vi "measureCombs_anySet2.vi"(3 "Read freqs. \nfrom textfile":bool, 5 "Cluster":T2={"span"=200000000.0, "rbw"=1000.0, "enableVBW"=FALSE, "vbw"=0.0, "traceLength"=64001, "window"=0, "verticalUnit"=0, "center freq"=100000000.0} {"verticalUnit" items=["SpectrumVerticalUnit_dBm", "SpectrumVerticalUnit_Watt", "SpectrumVerticalUnit_Volt", "SpectrumVerticalUnit_Amp", "SpectrumVerticalUnit_dBmV"]; "window" items=["SpectrumWindow_Kaiser", "SpectrumWindow_Mil6dB", "SpectrumWindow_BlackmanHarris", "SpectrumWindow_Rectangle", "SpectrumWindow_FlatTop", "SpectrumWindow_Hann"]; "traceLength" items=["801"=801, "2401"=2401, "4001"=4001, "8001"=8001, "10401"=10401, "16001"=16001, "32001"=32001, "64001"=64001]}, 6 "error in":errorcluster, 7 "Burn time/ RFC measurement time":i32=2, 8 "AFC & OFC Measurement time":i32=2, 9 "Folder for all data (Don't forget the last slash!)":string="C:\\Users\\Lab\\Desktop\\Data\\2019-08\\2019-08-07\\") -> (0 "error out":errorcluster)   [LabVIEW 2016]
uses:
  <vilib>/Utility/file.llb/Read Delimited Spreadsheet (DBL).vi
  <vilib>/Utility/file.llb/Write Delimited Spreadsheet (DBL).vi
panel:
  in  "stop":bool
  out "error out 2":errorcluster
  out "traceData out":sgl[](graph)
  out "To change these settings, you must edit them in the block diagram":T1(array[cluster])
  in  "Sweep probe twice":bool
  out "Current set #":i32
  out "Current freq.":dbl
  in  "freqs. file":path
  in  "Shuffle?":bool
  in  "Start freq":dbl=1000000.0 format="%0.2e"
  in  "End freq":dbl=2000000.0 format="%0.2e"
  in  "Freq step":i32=100000 format="%.2e"
  out "Duration array":T3(array[cluster])
  in  "Mod shape":enum16{"Triangle", "Sine"}(ring)
  # "consecutive sweeps can be compared\nto check for probe on AFC."
  # "RSA settings"
  # "Suppose you want to collect comb data, first ascending, then descending.\n\nIn Matlab, create a 1xM array \ncontaining all modulation freqs (Hz) in the ascending sequence; then create a 1xN array for the descending case. Note that M != N is fine.\n\nfid= fopen(FILENAME, 'w');\nfprintf(fid,'%d\\t', ARRAY1);\nfprintf(fid,'\\r\\n');\nfprintf(fid,'%d\\t',ARRAY2);\n... \n(for more sets, repeat as needed)\nfclose(fid);\n\nNow find the file you just made:"
  # "Modulation settings"
  # "(zero-indexed)"
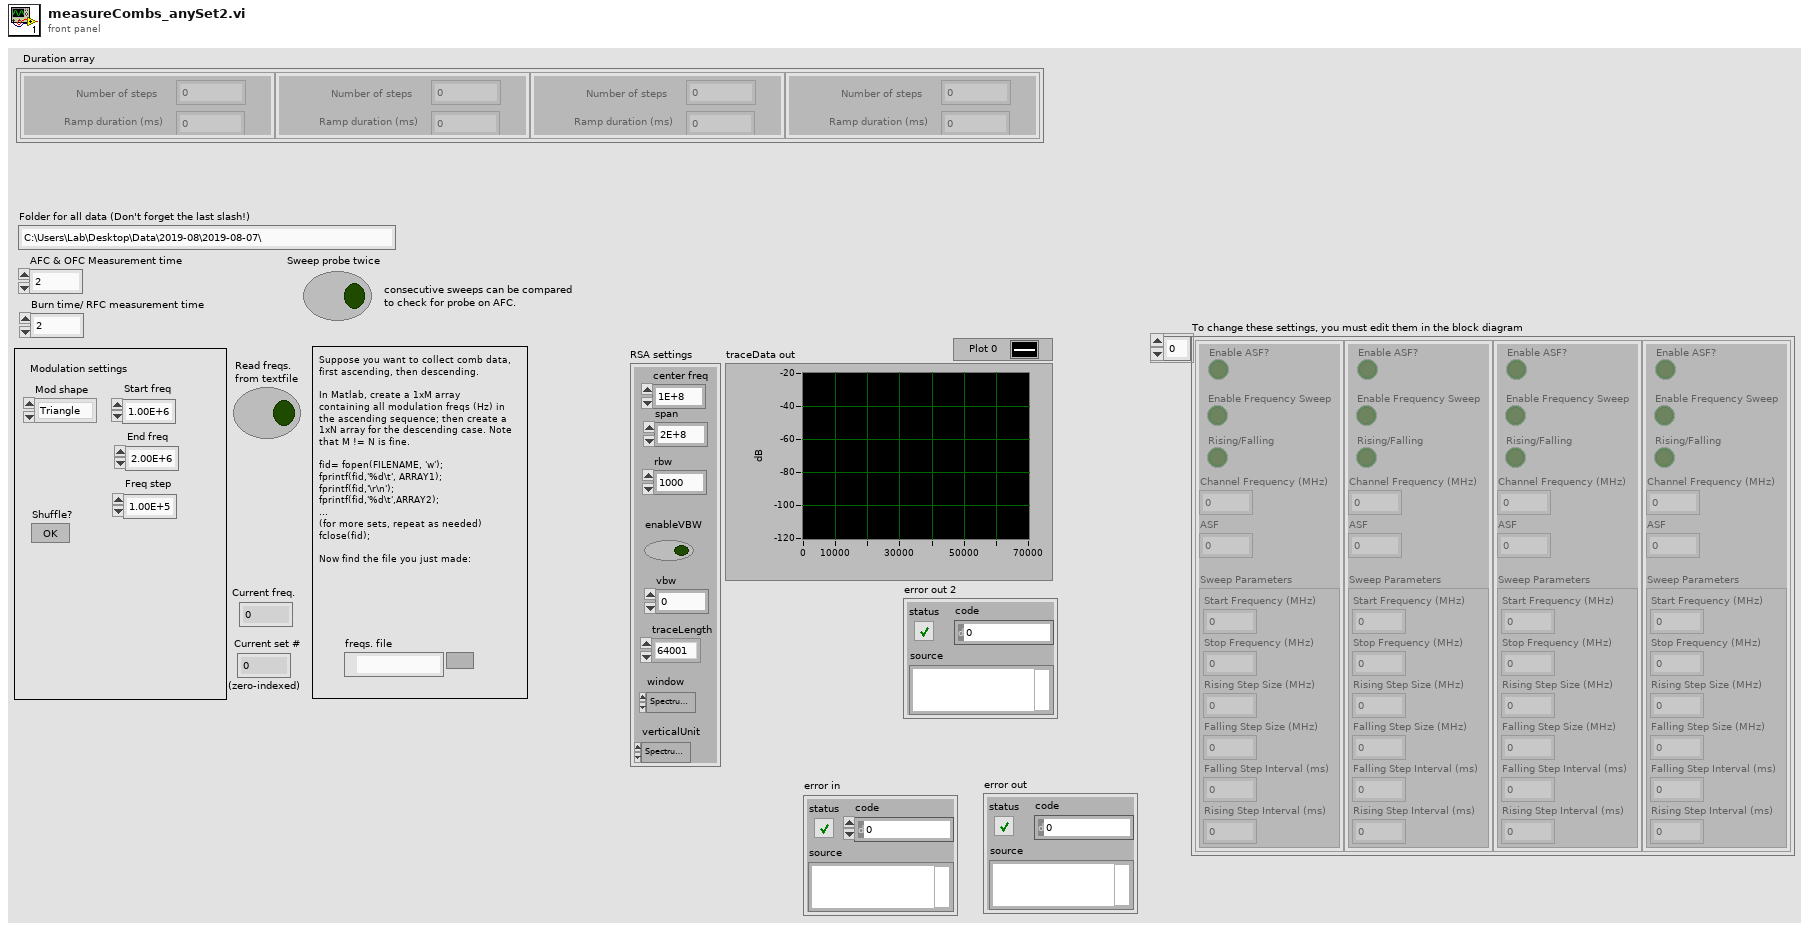
[diagram p1: front panel]
types:
  T1 = cluster{"Enable ASF?":bool, "Channel Frequency (MHz)":dbl, "ASF":dbl, "Enable Frequency Sweep":bool, "Sweep Parameters":cluster{"Start Frequency (MHz)":dbl, "Stop Frequency (MHz)":dbl, "Rising Step Size (MHz)":dbl, "Falling Step Size (MHz)":dbl, "Falling Step Interval (ms)":dbl, "Rising Step Interval (ms)":dbl}, "Rising/Falling":bool}[]
  T2 = cluster{"span":dbl, "rbw":dbl, "enableVBW":bool, "vbw":dbl, "traceLength":u16, "window":u32, "verticalUnit":u32, "center freq":dbl}
  T3 = cluster{"Number of steps":dbl, "Ramp duration (ms)":dbl}[]
  T4 = cluster{"span":dbl, "rbw":dbl, "enableVBW":bool, "vbw":dbl, "traceLength":u16, "window":u32, "verticalUnit":u32}
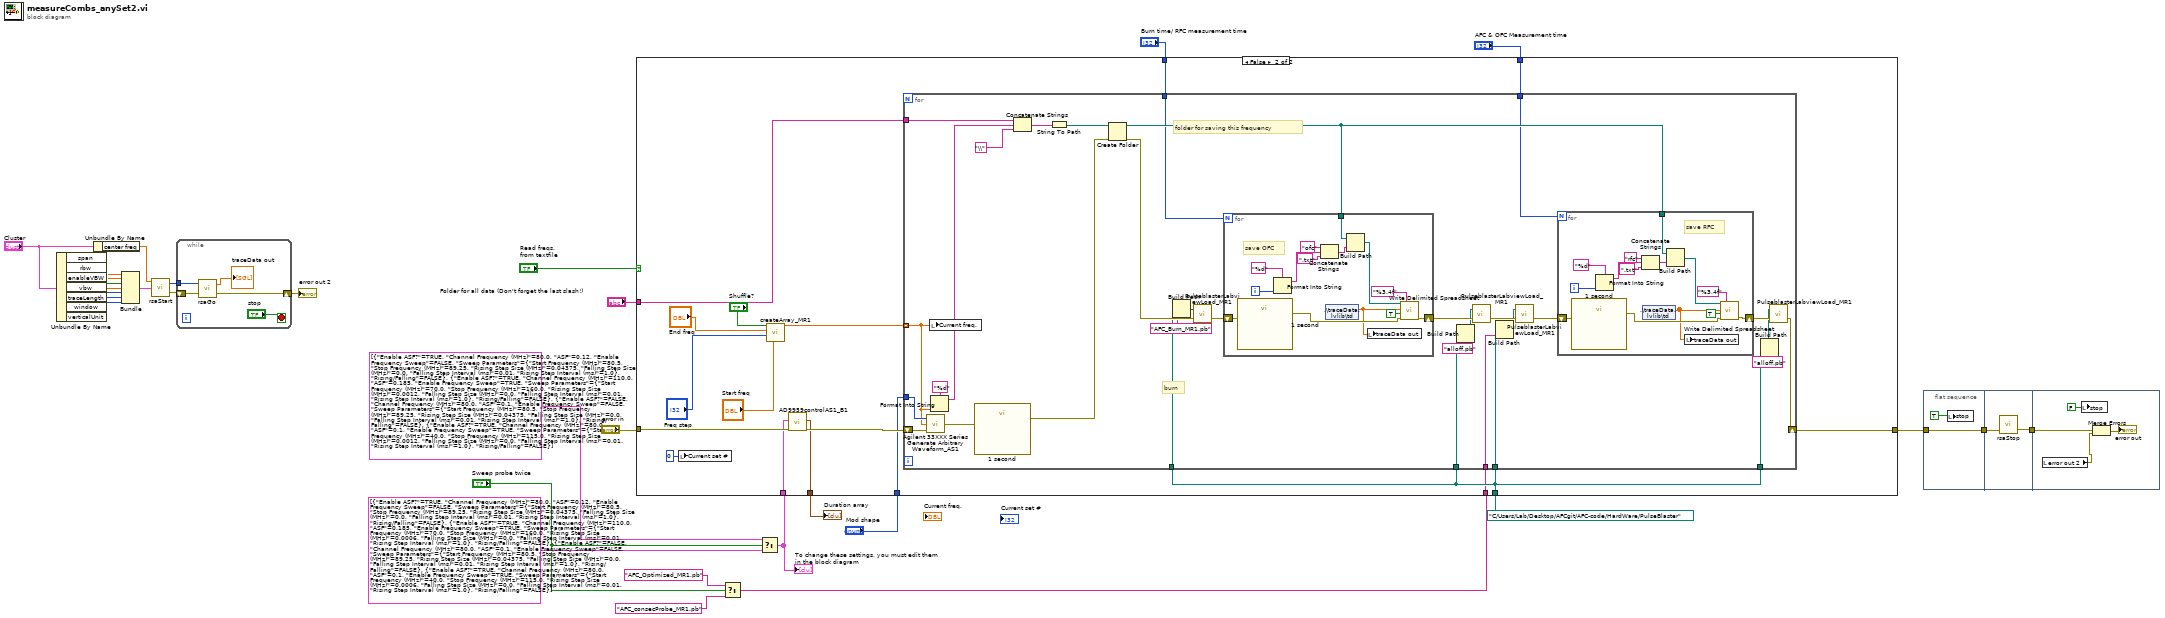
[diagram p0: block diagram]
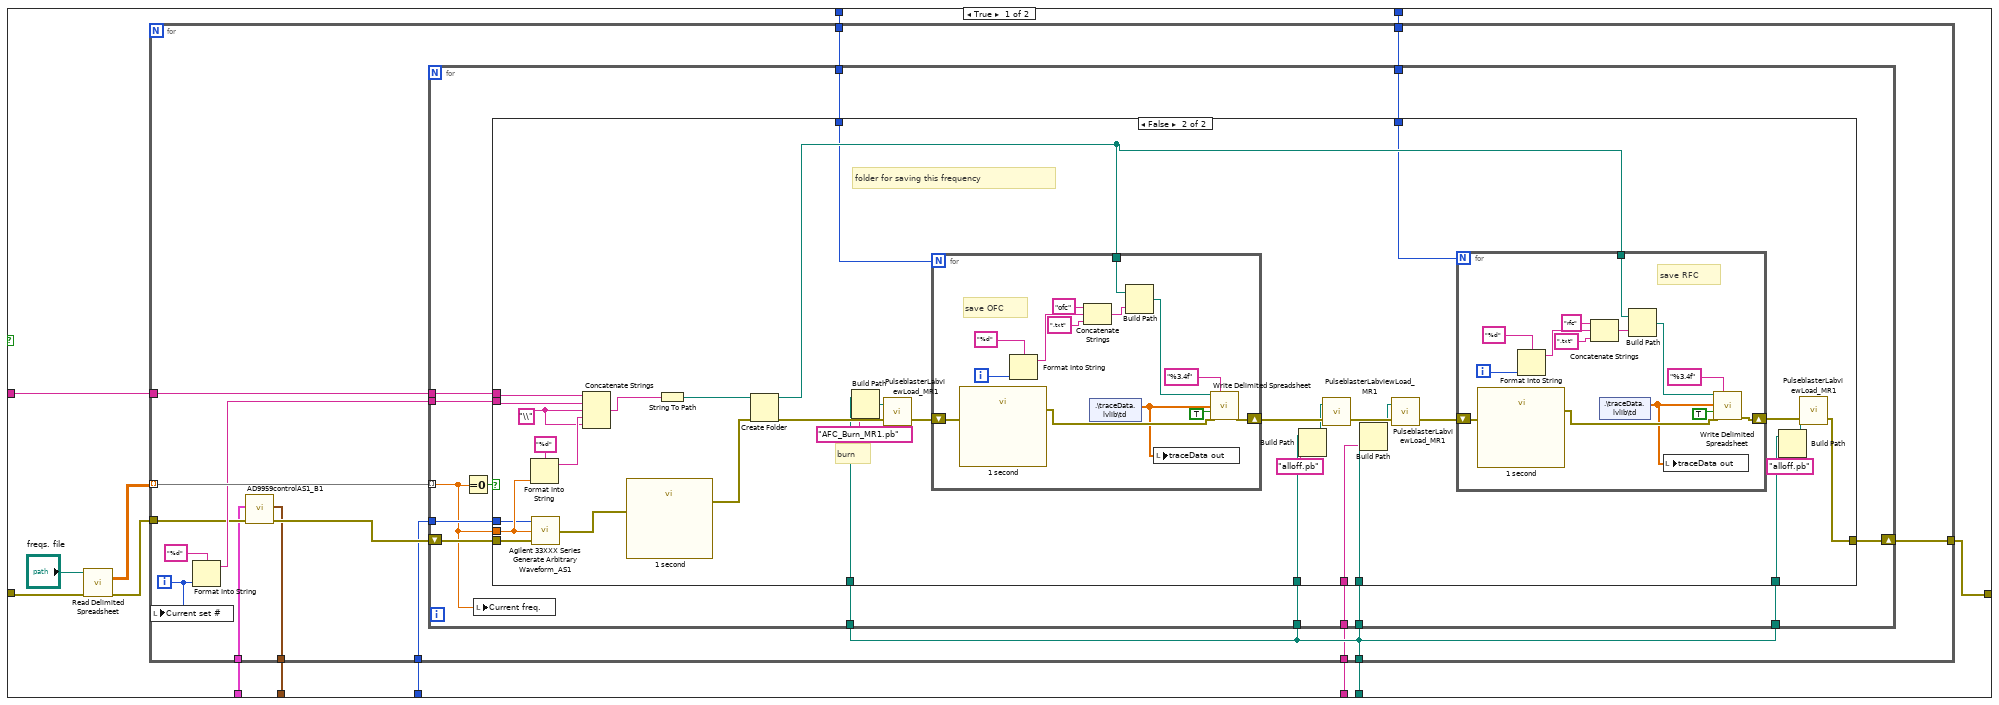
[diagram p2: hidden frame]
diagram:
  n1 = Unbundle By Name("Cluster") -> ("span"=w24:dbl, "rbw"=w25:dbl, "enableVBW"=w26:bool, "vbw"=w27:dbl, "traceLength"=w28:u16, "window"=w29:u32, "verticalUnit"=w30:u32)
  n2 = Unbundle By Name("Cluster") -> ("center freq"=w7:dbl)
  n3 = Bundle("span"=w24, "rbw"=w25, "enableVBW"=w26, "vbw"=w27, "traceLength"=w28, "window"=w29, "verticalUnit"=w30) -> (w6:T4)  [unwired: 1 in]
  n4 = call "rsaStart.vi"("Cluster"=w6, "center freq"=w7) -> ("error out"=w4:errorcluster, "traceLength"=w5:u16)  [unwired: 1 in]
  n5 = while {
    tunnel: w5 -> [w36]
    shift-right: [w34] -> w3
    shift-left: w4 -> [w33]
    stop <- "stop" stop-if-true
    n6 = call "rsaGo.vi"("error in"=w33, "Trace length"=w36) -> ("error out"=w34:errorcluster, "traceData out"=→"traceData out":sgl[])  [unwired: 1 in]
  }
  "error out 2" <- w3
  n7 = Select(t="AFC_Optimized_MR1.pb" ("name or relative path"), s="Sweep probe twice", f="AFC_consecProbe_MR1.pb" ("name or relative path")) -> (s? t:f=w8:string)
  n8 = Select(t=T1 [{"Enable ASF?"=TRUE, "Channel Frequency (MHz)"=80.0, "ASF"=0.12, "Enable Frequency Sweep"=FALSE, "Sweep Parameters"={"Start Frequency (MHz)"=80.5, "Stop Frequency (MHz)"=89.25, "Rising Step Size (MHz)"=0.04375, "Falling Step Size (MHz)"=0.0, "Falling Step Interval (ms)"=0.01, "Rising Step Interval (ms)"=1.0}, "Rising/Falling"=FALSE}, {"Enable ASF?"=TRUE, "Channel Frequency (MHz)"=110.0, "ASF"=0.185, "Enable Frequency Sweep"=TRUE, "Sweep Parameters"={"Start Frequency (MHz)"=70.0, "Stop Frequency (MHz)"=160.0, "Rising Step Size (MHz)"=0.0012, "Falling Step Size (MHz)"=0.0, "Falling Step Interval (ms)"=0.01, "Rising Step Interval (ms)"=1.0}, "Rising/Falling"=FALSE}, {"Enable ASF?"=FALSE, "Channel Frequency (MHz)"=80.0, "ASF"=0.1, "Enable Frequency Sweep"=FALSE, "Sweep Parameters"={"Start Frequency (MHz)"=80.5, "Stop Frequency (MHz)"=89.25, "Rising Step Size (MHz)"=0.04375, "Falling Step Size (MHz)"=0.0, "Falling Step Interval (ms)"=0.01, "Rising Step Interval (ms)"=1.0}, "Rising/Falling"=FALSE}, {"Enable ASF?"=TRUE, "Channel Frequency (MHz)"=80.0, "ASF"=0.1, "Enable Frequency Sweep"=TRUE, "Sweep Parameters"={"Start Frequency (MHz)"=40.0, "Stop Frequency (MHz)"=115.0, "Rising Step Size (MHz)"=0.0012, "Falling Step Size (MHz)"=0.0, "Falling Step Interval (ms)"=0.01, "Rising Step Interval (ms)"=1.0}, "Rising/Falling"=FALSE}] ("Array"), s="Sweep probe twice", f=T1 [{"Enable ASF?"=TRUE, "Channel Frequency (MHz)"=80.0, "ASF"=0.12, "Enable Frequency Sweep"=FALSE, "Sweep Parameters"={"Start Frequency (MHz)"=80.5, "Stop Frequency (MHz)"=89.25, "Rising Step Size (MHz)"=0.04375, "Falling Step Size (MHz)"=0.0, "Falling Step Interval (ms)"=0.01, "Rising Step Interval (ms)"=1.0}, "Rising/Falling"=FALSE}, {"Enable ASF?"=TRUE, "Channel Frequency (MHz)"=110.0, "ASF"=0.185, "Enable Frequency Sweep"=TRUE, "Sweep Parameters"={"Start Frequency (MHz)"=70.0, "Stop Frequency (MHz)"=160.0, "Rising Step Size (MHz)"=0.0006, "Falling Step Size (MHz)"=0.0, "Falling Step Interval (ms)"=0.01, "Rising Step Interval (ms)"=1.0}, "Rising/Falling"=FALSE}, {"Enable ASF?"=FALSE, "Channel Frequency (MHz)"=80.0, "ASF"=0.1, "Enable Frequency Sweep"=FALSE, "Sweep Parameters"={"Start Frequency (MHz)"=80.5, "Stop Frequency (MHz)"=89.25, "Rising Step Size (MHz)"=0.04375, "Falling Step Size (MHz)"=0.0, "Falling Step Interval (ms)"=0.01, "Rising Step Interval (ms)"=1.0}, "Rising/Falling"=FALSE}, {"Enable ASF?"=TRUE, "Channel Frequency (MHz)"=80.0, "ASF"=0.1, "Enable Frequency Sweep"=TRUE, "Sweep Parameters"={"Start Frequency (MHz)"=40.0, "Stop Frequency (MHz)"=115.0, "Rising Step Size (MHz)"=0.0006, "Falling Step Size (MHz)"=0.0, "Falling Step Interval (ms)"=0.01, "Rising Step Interval (ms)"=1.0}, "Rising/Falling"=FALSE}] ("Array")) -> (s? t:f=w12:T1)
  "To change these settings, you must edit them in the block diagram" <- w12
  n9 = case shown="False" "Read freqs. \nfrom textfile" {
    tunnel: "Folder for all data (Don't forget the last slash!)" -> [w49 w158]
    tunnel: path "C:/Users/Lab/Desktop/AFCgit/AFC-code/HardWare/PulseBlaster" ("base path") -> [w39 w157]
    tunnel: "Burn time/ RFC measurement time" -> [w48 w155]
    tunnel: "AFC & OFC Measurement time" -> [w47 w154]
    tunnel: "error in" -> [w45 w148]
    tunnel: "Mod shape" -> [w42 w147]
    tunnel: w12 -> [w41 w146]
    tunnel: [w40 w145] -> w15
    tunnel: w8 -> [w38 w143]
    tunnel: [w37 w142] -> w31
    frame True {
      n10 = call-poly <vilib>:"Read Delimited Spreadsheet.vi"("file path (dialog if empty)"="freqs. file", "error in (no error)"=w45) -> ("all rows"=w44:dbl[][], "error out"=w43:errorcluster)  [unwired: 8 in, 4 out]
      n11 = for {
        tunnel: [w64] -> w37
        tunnel: w49 -> [w63]
        tunnel: w39 -> [w62]
        tunnel: w48 -> [w60]
        tunnel: w47 -> [w59]
        tunnel: w44 -> [w58] mode=indexing
        tunnel: w43 -> [w55]
        tunnel: w42 -> [w54]
        tunnel: w41 -> [w53]
        tunnel: [w52] -> w40
        tunnel: w38 -> [w50]
        i -> [w51]
        n12 = local write "Current set #"(w51) -> ()
        n13 = Format Into String(format string="%d", w51) -> (resulting string=w56:string)  [unwired: 2 in, 1 out]
        n14 = call "AD9959controlAS1_B1.vi"("error in (no error)"=w55, "Array"=w53) -> ("error out"=w61:errorcluster, "Duration array"=w52:T3)  [unwired: 8 in]
        n15 = for {
          tunnel: w58 -> [w66] mode=indexing
          tunnel: w54 -> [w78]
          shift-right: [w77] -> w64
          shift-left: w61 -> [w76]
          tunnel: w63 -> [w68]
          tunnel: w62 -> [w75]
          tunnel: w62 -> [w74]
          tunnel: w62 -> [w73]
          tunnel: w62 -> [w72]
          tunnel: w60 -> [w71]
          tunnel: w59 -> [w70]
          tunnel: w56 -> [w69]
          tunnel: w50 -> [w65]
          n16 = Equal To 0?(x=w66) -> (x = 0?=w67:bool)
          n17 = local write "Current freq."(w66) -> ()
          n18 = case shown="False" w67 {
            tunnel: w78 -> [_ w81]
            tunnel: [w79 w113] -> w77
            tunnel: w76 -> [w79 w83]
            tunnel: w75 -> [_ w102]
            tunnel: w74 -> [_ w99]
            tunnel: w73 -> [_ w97]
            tunnel: w72 -> [_ w94]
            tunnel: w71 -> [_ w92]
            tunnel: w70 -> [_ w91]
            tunnel: w69 -> [_ w86]
            tunnel: w68 -> [_ w87]
            tunnel: w66 -> [_ w82]
            tunnel: w65 -> [_ w80]
            frame True {
            }
            frame False {
              w89 = "\\" ("string")
              # "folder for saving this frequency"
              # "burn"
              n19 = Format Into String(format string="%d", w82) -> (resulting string=w90:string)  [unwired: 2 in, 1 out]
              n20 = call "Agilent 33XXX Series Generate Arbitrary Waveform_AS1.vi"("error in (no error)"=w83, "Frequency (1000 Hz)"=w82, "Enum"=w81) -> ("error out"=w84:errorcluster)
              n21 = Concatenate Strings(w87, w86, w89, w90, w89) -> (w85:string)
              n22 = call "1 second"("error in (no error)"=w84) -> ("error out"=w106:errorcluster)  [unwired: 10 in]
              n23 = String To Path(string=w85) -> (path=w103:path)
              n24 = Create Folder(path (use dialog)=w103, error in=w106) -> (created path=w104:path, error out=w105:errorcluster)  [unwired: 1 in, 1 out]
              n25 = Build Path(base path=w102, name or relative path="AFC_Burn_MR1.pb") -> (appended path=w100:path)
              n26 = call "PulseblasterLabviewLoad_MR1.vi"("error in (no error)"=w105, "Input file"=w100) -> ("error out"=w112:errorcluster)  [unwired: 1 out]
              n27 = for {
                N: w92 -> [_]
                shift-right: [w140] -> w107
                shift-left: w112 -> [w130]
                tunnel: w104 -> [w133]
                i -> [w131]
                # "save OFC"
                n28 = call "1 second"("error in (no error)"=w130) -> ("error out"=w129:errorcluster)  [unwired: 10 in]
                n29 = Format Into String(format string="%d", w131) -> (resulting string=w136:string)  [unwired: 2 in, 1 out]
                n30 = Concatenate Strings("ofc" ("string"), w136, ".txt" ("string")) -> (w135:string)
                n31 = shared-variable ".\\traceData.lvlib\\td"() -> (w128:dbl[])  [unwired: 1 in, 1 out]
                n32 = Build Path(base path=w133, name or relative path=w135) -> (appended path=w139:path)
                n33 = local write "traceData out"(w128) -> ()
                n34 = call-poly <vilib>:"Write Delimited Spreadsheet.vi"("file path (dialog if empty)"=w139, "format (%.3f)"="%3.4f", "1D data"=w128, "append to file? (new file:F)"=TRUE, "error in (no error)"=w129) -> ("error out"=w140:errorcluster)  [unwired: 9 in, 1 out]
              }
              n35 = Build Path(base path=w97, name or relative path="alloff.pb") -> (appended path=w96:path)
              n36 = call "PulseblasterLabviewLoad_MR1.vi"("error in (no error)"=w107, "Input file"=w96) -> ("error out"=w108:errorcluster)  [unwired: 1 out]
              n37 = Build Path(base path=w99, name or relative path=w80) -> (appended path=w98:path)
              n38 = call "PulseblasterLabviewLoad_MR1.vi"("error in (no error)"=w108, "Input file"=w98) -> ("error out"=w110:errorcluster)  [unwired: 1 out]
              n39 = for {
                N: w91 -> [_]
                shift-right: [w126] -> w109
                shift-left: w110 -> [w116]
                tunnel: w104 -> [w118]
                i -> [w122]
                # "save RFC"
                n40 = call "1 second"("error in (no error)"=w116) -> ("error out"=w115:errorcluster)  [unwired: 10 in]
                n41 = Format Into String(format string="%d", w122) -> (resulting string=w121:string)  [unwired: 2 in, 1 out]
                n42 = Concatenate Strings("rfc" ("string"), w121, ".txt" ("string")) -> (w120:string)
                n43 = shared-variable ".\\traceData.lvlib\\td"() -> (w114:dbl[])  [unwired: 1 in, 1 out]
                n44 = Build Path(base path=w118, name or relative path=w120) -> (appended path=w125:path)
                n45 = local write "traceData out"(w114) -> ()
                n46 = call-poly <vilib>:"Write Delimited Spreadsheet.vi"("file path (dialog if empty)"=w125, "format (%.3f)"="%3.4f", "1D data"=w114, "append to file? (new file:F)"=TRUE, "error in (no error)"=w115) -> ("error out"=w126:errorcluster)  [unwired: 9 in, 1 out]
              }
              n47 = Build Path(base path=w94, name or relative path="alloff.pb") -> (appended path=w93:path)
              n48 = call "PulseblasterLabviewLoad_MR1.vi"("error in (no error)"=w109, "Input file"=w93) -> ("error out"=w113:errorcluster)  [unwired: 1 out]
            }
          }
        }
      }
    }
    frame False {
      n49 = local write "Current set #"(0 ("Current set #")) -> ()
      n50 = call "createArray_MR1.vi"("Start freq"="Start freq", "Freq step"="Freq step", "End freq"="End freq", "Shuffle?"="Shuffle?") -> ("Riffled {X}"=w149:dbl[])  [unwired: 7 in]
      n51 = call "AD9959controlAS1_B1.vi"("error in (no error)"=w148, "Array"=w146) -> ("error out"=w156:errorcluster, "Duration array"=w145:T3)  [unwired: 8 in]
      n52 = for {
        tunnel: w149 -> [w161] mode=indexing
        tunnel: w147 -> [w191]
        shift-right: [w190] -> w142
        shift-left: w156 -> [w189]
        tunnel: w158 -> [w164]
        tunnel: w157 -> [w174]
        tunnel: w157 -> [w171]
        tunnel: w157 -> [w169]
        tunnel: w157 -> [w166]
        tunnel: w155 -> [w163]
        tunnel: w154 -> [w162]
        tunnel: w143 -> [w160]
        # "folder for saving this frequency"
        # "burn"
        n53 = call "Agilent 33XXX Series Generate Arbitrary Waveform_AS1.vi"("error in (no error)"=w189, "Frequency (1000 Hz)"=w161, "Enum"=w191) -> ("error out"=w184:errorcluster)
        n54 = local write "Current freq."(w161) -> ()
        n55 = Format Into String(format string="%d", w161) -> (resulting string=w186:string)  [unwired: 2 in, 1 out]
        n56 = call "1 second"("error in (no error)"=w184) -> ("error out"=w179:errorcluster)  [unwired: 10 in]
        n57 = Concatenate Strings(w164, w186, "\\" ("string")) -> (w176:string)
        n58 = String To Path(string=w176) -> (path=w175:path)
        n59 = Create Folder(path (use dialog)=w175, error in=w179) -> (created path=w177:path, error out=w178:errorcluster)  [unwired: 1 in, 1 out]
        n60 = Build Path(base path=w174, name or relative path="AFC_Burn_MR1.pb") -> (appended path=w172:path)
        n61 = call "PulseblasterLabviewLoad_MR1.vi"("error in (no error)"=w178, "Input file"=w172) -> ("error out"=w188:errorcluster)  [unwired: 1 out]
        n62 = for {
          N: w163 -> [_]
          shift-right: [w218] -> w180
          shift-left: w188 -> [w208]
          tunnel: w177 -> [w211]
          i -> [w209]
          # "save OFC"
          n63 = call "1 second"("error in (no error)"=w208) -> ("error out"=w207:errorcluster)  [unwired: 10 in]
          n64 = Format Into String(format string="%d", w209) -> (resulting string=w214:string)  [unwired: 2 in, 1 out]
          n65 = Concatenate Strings("ofc" ("string"), w214, ".txt" ("string")) -> (w213:string)
          n66 = shared-variable ".\\traceData.lvlib\\td"() -> (w206:dbl[])  [unwired: 1 in, 1 out]
          n67 = Build Path(base path=w211, name or relative path=w213) -> (appended path=w217:path)
          n68 = local write "traceData out"(w206) -> ()
          n69 = call-poly <vilib>:"Write Delimited Spreadsheet.vi"("file path (dialog if empty)"=w217, "format (%.3f)"="%3.4f", "1D data"=w206, "append to file? (new file:F)"=TRUE, "error in (no error)"=w207) -> ("error out"=w218:errorcluster)  [unwired: 9 in, 1 out]
        }
        n70 = Build Path(base path=w169, name or relative path="alloff.pb") -> (appended path=w168:path)
        n71 = call "PulseblasterLabviewLoad_MR1.vi"("error in (no error)"=w180, "Input file"=w168) -> ("error out"=w181:errorcluster)  [unwired: 1 out]
        n72 = Build Path(base path=w171, name or relative path=w160) -> (appended path=w170:path)
        n73 = call "PulseblasterLabviewLoad_MR1.vi"("error in (no error)"=w181, "Input file"=w170) -> ("error out"=w183:errorcluster)  [unwired: 1 out]
        n74 = for {
          N: w162 -> [_]
          shift-right: [w204] -> w182
          shift-left: w183 -> [w194]
          tunnel: w177 -> [w196]
          i -> [w200]
          # "save RFC"
          n75 = call "1 second"("error in (no error)"=w194) -> ("error out"=w193:errorcluster)  [unwired: 10 in]
          n76 = Format Into String(format string="%d", w200) -> (resulting string=w199:string)  [unwired: 2 in, 1 out]
          n77 = Concatenate Strings("rfc" ("string"), w199, ".txt" ("string")) -> (w198:string)
          n78 = shared-variable ".\\traceData.lvlib\\td"() -> (w192:dbl[])  [unwired: 1 in, 1 out]
          n79 = Build Path(base path=w196, name or relative path=w198) -> (appended path=w203:path)
          n80 = local write "traceData out"(w192) -> ()
          n81 = call-poly <vilib>:"Write Delimited Spreadsheet.vi"("file path (dialog if empty)"=w203, "format (%.3f)"="%3.4f", "1D data"=w192, "append to file? (new file:F)"=TRUE, "error in (no error)"=w193) -> ("error out"=w204:errorcluster)  [unwired: 9 in, 1 out]
        }
        n82 = Build Path(base path=w166, name or relative path="alloff.pb") -> (appended path=w165:path)
        n83 = call "PulseblasterLabviewLoad_MR1.vi"("error in (no error)"=w182, "Input file"=w165) -> ("error out"=w190:errorcluster)  [unwired: 1 out]
      }
    }
  }
  "Duration array" <- w15
  n84 = flat-sequence {
    tunnel: w31 -> [w221]
    tunnel: [w221] -> w2
    tunnel: w2 -> [w223]
    tunnel: [w222] -> w1
    tunnel: w1 -> [w227]
    frame #0 {
      n85 = local write "stop"(TRUE ("Stop")) -> ()
    }
    frame #1 {
      n86 = call "rsaStop.vi"("error in (no error)"=w223) -> ("error out"=w222:errorcluster)  [unwired: 3 in]
    }
    frame #2 {
      n87 = local read "error out 2"() -> (w226:errorcluster)
      n88 = local write "stop"(FALSE ("stop")) -> ()
      n89 = Merge Errors(w227, w226) -> (→"error out":errorcluster)
    }
  }
